vi "countrate.vi"() -> ()   [LabVIEW 2015]
uses:
  <vilib>/Platform/TimedLoop/XDataNode/timing_clust.ctl
  <vilib>/Platform/TimedLoop/XDataNode/nitl_modes.ctl
  <vilib>/Platform/TimedLoop/XDataNode/wakeup.ctl
  <vilib>/imath/engines/lvmath2/RunTimeEngine/Managers/WorkSpace/UID Generator.vi
  <vilib>/imath/engines/lvmath2/RunTimeEngine/RangeToken/NIMS_Range.vi
  <instcachedir>/0/NIMS_Range_D919CC09935940E88F755EC1C6F49AC1.lvgen/NIMS_Range_D919CC09935940E88F755EC1C6F49AC1_000.vi
  <vilib>/imath/engines/lvmath2/RunTimeEngine/RunTimeType/NIMS_RunTimeType_From StrictType (excl LVString).vi
  <instcachedir>/0/NIMS_RunTimeType_From StrictType (excl LVString)_EB1C38A9BC5048DA9ABDA8F781E54D21.lvgen/NIMS_RunTimeType_From StrictType (excl LVString)_EB1C38A9BC5048DA9ABDA8F781E54D21_000.vi
  <vilib>/imathl/engines/lvmath/Functions/Error Handling/Create Error.vi
  <vilib>/imath/engines/lvmath2/RunTimeEngine/LocalVariableDefStatement/MC_LocalVariableDefStatement_Display.vi
  <vilib>/imath/engines/lvmath2/RunTimeEngine/Managers/SymbolTable/Clear UID.vi
  <vilib>/imath/engines/lvmath2/RunTimeEngine/NodeEndStatement/NIMS_NodeEndStatement_Output.vi
  <instcachedir>/0/NIMS_NodeEndStatement_Output_53EC0D466D134D7ABD903AC30B43404B.lvgen/NIMS_NodeEndStatement_Output_53EC0D466D134D7ABD903AC30B43404B_005.vi
  <vilib>/imath/engines/lvmath2/RunTimeEngine/ErrorHandling/NIMS_Finalize Error.vi
  <vilib>/Utility/file.llb/Write Delimited Spreadsheet (DBL).vi
  <vilib>/platform/TimedLoop/XDataNode/XDataNode.xnode
  <vilib>/Platform/TimedLoop/XDataNode/XDNodeRunTimeDep.lvlib
  <vilib>/imath/engines/lvmath2/RunTimeEngine/Managers/SymbolTable/NIMS_WorkSpace.lvlib
panel:
  out "XY Graph":cluster{"t":dbl[], i32[]}(graph)={"t"=[0.0, 1.0, 2.0, 3.0, 4.0, 5.0, 6.0, 7.0, 8.0, 9.0, 10.0, 11.0, 12.0, 13.0, 14.0, 15.0, 16.0, 17.0, 18.0, 19.0, 20.0, 21.0, 22.0, 23.0, 24.0, 25.0, 26.0, 27.0, 28.0, 29.0, 30.0, 31.0, 32.0, 33.0, 34.0, 35.0, 36.0, 37.0, 38.0, 39.0, 40.0, 41.0, 42.0, 43.0, 44.0, 45.0, 46.0, 47.0, 48.0, 49.0, 50.0, 51.0, 52.0, 53.0, 54.0, 55.0, 56.0, 57.0, 58.0, 59.0, 60.0, 61.0, 62.0, 63.0, 64.0, 65.0, 66.0, 67.0, 68.0, 69.0, 70.0, 71.0, 72.0, 73.0, 74.0, 75.0, 76.0, 77.0, 78.0, 79.0, 80.0, 81.0, 82.0, 83.0, 84.0, 85.0, 86.0, 87.0, 88.0, 89.0, 90.0, 91.0, 92.0, 93.0, 94.0, 95.0, 96.0, 97.0, 98.0, 99.0, 100.0, 101.0, 102.0, 103.0, 104.0, 105.0, 106.0, 107.0, 108.0, 109.0, 110.0, 111.0, 112.0, 113.0, 114.0, 115.0, 116.0, 117.0, 118.0, 119.0, 120.0, 121.0, 122.0, 123.0, 124.0, 125.0, 126.0, 127.0, 128.0, 129.0, 130.0, 131.0, 132.0, 133.0, 134.0, 135.0, 136.0, 137.0, 138.0, 139.0, 140.0, 141.0, 142.0, 143.0, 144.0, 145.0, 146.0, 147.0, 148.0, 149.0, 150.0, 151.0, 152.0, 153.0, 154.0, 155.0, 156.0, 157.0, 158.0, 159.0, 160.0, 161.0, 162.0, 163.0, 164.0, 165.0, 166.0, 167.0, 168.0, 169.0, 170.0, 171.0, 172.0, 173.0, 174.0, 175.0, 176.0, 177.0, 178.0, 179.0, 180.0, 181.0, 182.0, 183.0, 184.0, 185.0, 186.0, 187.0, 188.0, 189.0, 190.0, 191.0, 192.0, 193.0, 194.0, 195.0, 196.0, 197.0, 198.0, 199.0, 200.0, 201.0, 202.0, 203.0, 204.0, 205.0, 206.0, 207.0, 208.0, 209.0, 210.0, 211.0, 212.0, 213.0, 214.0, 215.0, 216.0, 217.0, 218.0, 219.0, 220.0, 221.0, 222.0, 223.0, 224.0, 225.0, 226.0, 227.0, 228.0, 229.0, 230.0, 231.0, 232.0, 233.0, 234.0, 235.0, 236.0, 237.0, 238.0, 239.0, 240.0, 241.0, 242.0, 243.0, 244.0, 245.0, 246.0, 247.0, 248.0, 249.0, 250.0, 251.0, 252.0, 253.0, 254.0, 255.0, 256.0, 257.0, 258.0, 259.0, 260.0, 261.0, 262.0, 263.0, 264.0, 265.0, 266.0, 267.0, 268.0, 269.0, 270.0, 271.0, 272.0, 273.0, 274.0, 275.0, 276.0, 277.0, 278.0, 279.0, 280.0, 281.0, 282.0, 283.0, 284.0, 285.0, 286.0, 287.0, 288.0, 289.0, 290.0, 291.0, 292.0, 293.0, 294.0, 295.0, 296.0, 297.0, 298.0, 299.0, 300.0], [0, 52, 64, 47, 49, 52, 61, 57, 56, 66, 66, 65, 53, 61, 62, 39, 74, 65, 64, 64, 58, 49, 63, 47, 49, 42, 53, 54, 52, 47, 50, 37, 51, 49, 52, 51, 48, 50, 41, 47, 48, 49, 47, 59, 53, 42, 36, 35, 45, 45, 44, 60, 44, 38, 36, 37, 44, 28, 43, 37, 31, 37, 35, 33, 37, 34, 35, 29, 39, 31, 25, 34, 41, 30, 38, 34, 23, 32, 28, 36, 33, 37, 35, 26, 40, 33, 27, 28, 28, 25, 33, 29, 19, 25, 28, 34, 25, 28, 21, 27, 25, 32, 30, 20, 28, 27, 28, 28, 21, 24, 18, 23, 25, 22, 14, 24, 22, 32, 28, 28, 21, 34, 15, 20, 17, 20, 26, 26, 28, 19, 19, 16, 26, 18, 29, 22, 16, 20, 18, 22, 22, 16, 11, 13, 20, 20, 25, 15, 16, 15, 21, 16, 18, 8, 17, 18, 10, 13, 13, 21, 17, 11, 16, 17, 21, 15, 17, 17, 14, 17, 23, 15, 14, 12, 13, 9, 4, 21, 14, 17, 12, 22, 18, 8, 11, 8, 12, 14, 12, 26, 13, 12, 8, 13, 14, 12, 13, 11, 10, 11, 12, 12, 12, 11, 8, 14, 9, 7, 7, 8, 6, 13, 12, 14, 7, 11, 11, 8, 7, 6, 8, 11, 9, 9, 5, 6, 8, 6, 9, 10, 10, 5, 9, 6, 9, 8, 12, 7, 11, 7, 3, 7, 9, 9, 7, 13, 7, 9, 4, 13, 7, 6, 12, 10, 6, 12, 11, 4, 7, 10, 9, 8, 6, 5, 7, 10, 9, 9, 6, 8, 8, 4, 12, 8, 10, 3, 2, 4, 8, 9, 4, 2, 6, 5, 6, 8, 6, 6, 6, 6, 6, 3, 1, 6, 2, 4, 3, 4, 0, 4, 6]}
  in  "Run Time (min)":dbl=5.0
  in  "dt (s)":dbl=1.0
  out "counts per second":dbl(knob)=6.0 scale=0.0..100.0
  in  "stop":bool
  # "Demo count rate VI for Physics 434"
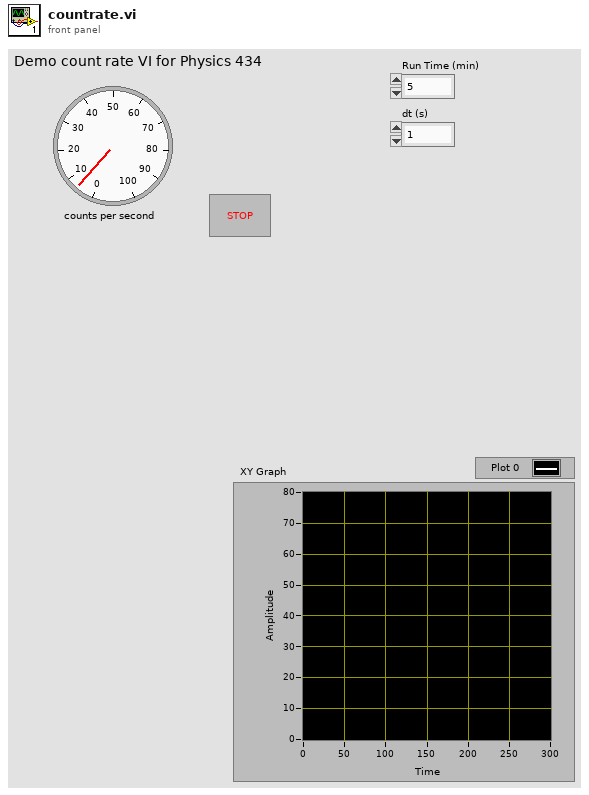
[diagram p1: front panel]
types:
  T1 = typedef "XDNodeRunTimeDep.lvlib/timing_clust.ctl" = cluster{"Expected End [f-1]":u64, "Actual End [f-1]":u64, "Finished Late? [f-1]":bool, "Expected End [i-1]":u64, "Actual End [i-1]":u64, "Finished Late? [i-1]":bool, "Expected Start [i]":u64, "Actual Start [i]":u64, "Expected Start [f]":u64, "Actual Start [f]":u64, "Source Name":string, "Structure Name":string, "Period":i64, "Deadline":i64, "Offset":i64, "Start":i64, "Priority":i32, "Timeout":i32, "Mode":T2, "Wakeup Reason":T3, "Error":errorcluster, "Source Type":string, "Secondary Source Type":string, "Global End Time":u64, "Global Start Time":u64, "Frame Duration":u64, "Iteration Duration":u64, "Assigned CPU":i32, "I/O Scan Engine Mode":u32}
  T2 = typedef "XDNodeRunTimeDep.lvlib/nitl_modes.ctl" = enum32{"No Change", "Process missed periods, maintain original phase", "Discard missed periods, maintain original phase", "Process missed periods, ignore original phase", "Discard missed periods, ignore original phase"}
  T3 = typedef "XDNodeRunTimeDep.lvlib/wakeup.ctl" = enum32{"Normal", "Aborted", "Asynchronous wakeup", "Timing source error", "Timed loop error", "Timeout"}
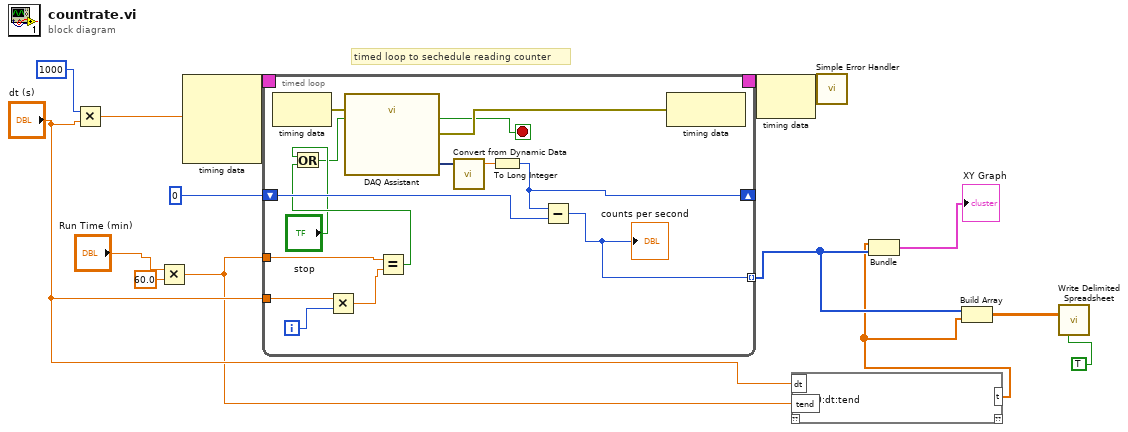
[diagram p0: block diagram]
diagram:
  # "timed loop to sechedule reading counter"
  n1 = Multiply(x=i64 1000 ("Period"), y="dt (s)") -> (x*y=w11:dbl)
  n2 = Multiply(x="Run Time (min)", y=60.0) -> (x*y=w1:dbl)
  n3 = node-c288(w11) -> (w15:T1)  [unwired: 3 in]
  n4 = timed-loop {
    timing: w15 -> [_]
    timing-out: [_] -> w14
    shift-right: [w21] -> _
    shift-left: 0 -> [w29]
    tunnel: "dt (s)" -> [w25]
    tunnel: w1 -> [w23]
    tunnel: [w16] -> w7 mode=indexing
    i -> [w22]
    stop <- w20 stop-if-true
    n5 = node-c288() -> (w26:errorcluster)  [unwired: 1 in]
    n6 = Multiply(x=w25, y=w22) -> (x*y=w24:dbl)
    n7 = Equal?(x=w23, y=w24) -> (x = y?=w19:bool)
    n8 = Or(x="stop", y=w19) -> (x .or. y?=w17:bool)
    n9 = call "DAQ Assistant"("error in"=w26, "stop (F)"=w17) -> ("data"=w30:dynamicdata, "stopped"=w20:bool, "error out"=w27:errorcluster)  [unwired: 14 in, 1 out]
    n10 = call "Convert from Dynamic Data"("Dynamic Data Type"=w30) -> ("Scalar"=w28:dbl)  [unwired: 3 in]
    n11 = To Long Integer(number=w28) -> (32bit integer=w21:i32)
    n12 = Subtract(x=w21, y=w29) -> (x-y=w16:i32)
    "counts per second" <- w16
    n13 = node-c288(w27) -> ()  [unwired: 1 out]
  }
  n14 = node-c288(w14) -> (w13:errorcluster)
  n15 = mathscript code="t =0:dt:tend"("dt"="dt (s)", "tend"=w1) -> ("t"=w6:dbl[])  [unwired: 1 in, 1 out]
  n16 = call <vilib>:"Simple Error Handler.vi"("error in (no error)"=w13) -> ()  [unwired: 4 in, 5 out]
  n17 = Bundle("t"=w6, w7) -> (→"XY Graph":cluster{"t":dbl[], i32[]})  [unwired: 1 in]
  n18 = Build Array(w7, w6) -> (w5:dbl[][])
  n19 = call-poly <vilib>:"Write Delimited Spreadsheet.vi"("2D data"=w5, "transpose? (F)"=TRUE) -> ()  [unwired: 12 in, 2 out]
